vi "GetOutState_ins.vi"(4 "error in":errorcluster, 5 "connection ID":refnum<k5>) -> (1 "error out":errorcluster, 2 "connection ID out":refnum<k5>, 3 "Answer":bool)   [LabVIEW 2013]
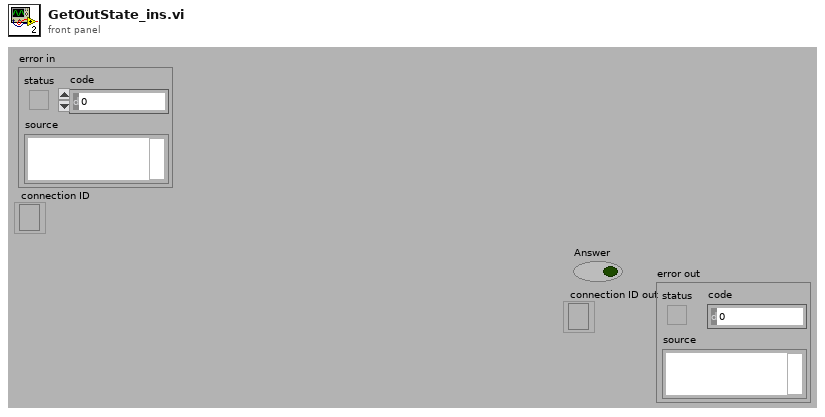
[diagram p1: front panel]
types:
  T1 = enum16{"Standard", "Buffered", "CRLF", "Immediate"}
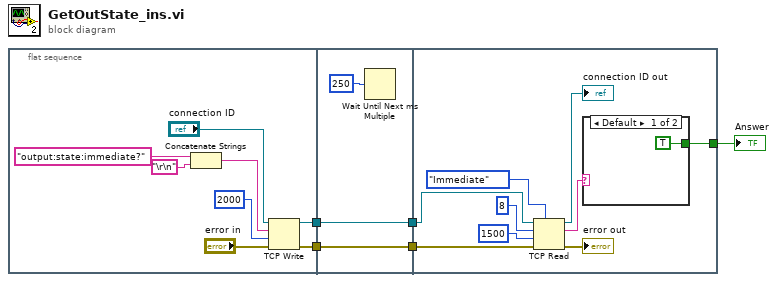
[diagram p0: block diagram]
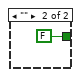
[diagram p2: hidden frame]
diagram:
  n1 = flat-sequence {
    tunnel: [w10] -> w4
    tunnel: [w9] -> w2
    tunnel: [w15] -> w5
    tunnel: w4 -> [w15]
    tunnel: [w14] -> w3
    tunnel: w2 -> [w14]
    tunnel: w5 -> [w19]
    tunnel: w3 -> [w18]
    tunnel: [w17] -> w1
    frame #0 {
      n2 = Concatenate Strings("output:state:immediate?" ("data in"), "\r\n") -> (w7:string)
      n3 = TCP Write(connection ID="connection ID", data in=w7, error in (no error)="error in", 9:2000 ("timeout ms (25000)")) -> (connection ID out=w10:refnum<k5>, error out=w9:errorcluster)  [unwired: 1 out]
    }
    frame #1 {
      n4 = Wait Until Next ms Multiple(millisecond multiple=u32 250) -> ()  [unwired: 1 out]
    }
    frame #2 {
      n5 = TCP Read(connection ID=w19, bytes to read=8, error in (no error)=w18, 7:T1."Immediate" ("mode (standard)"), 9:1500 ("timeout ms (25000)")) -> (connection ID out=→"connection ID out":refnum<k5>, data out=w23:string, error out=→"error out":errorcluster)
      n6 = case shown="Default" w23 {
        tunnel: [TRUE FALSE] -> w17
        frame Default {
        }
        frame "" {
        }
      }
    }
  }
  "Answer" <- w1
